vi "Correct Na-DAS_7609 sample interval error.vi"() -> ()   [LabVIEW 2022 SP3]
uses:
  Globals/Meas_global.vi
  Controls/Trigger_Mode.ctl
panel:
  out "Req Sample Rate Hz":dbl
  out "Delay Factor (s) per LDA sample":dbl
  in  "Apply time shift":bool=TRUE
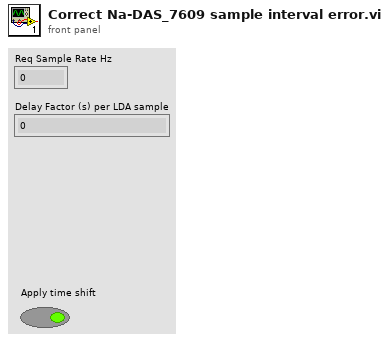
[diagram p1: front panel]
types:
  T1 = typedef "Time_Trace_Cluster.ctl" = cluster{"Weighting":dbl[], "Voltage":dbl[], "Eng Values":dbl[]}
  T2 = typedef "Trigger_Mode.ctl" = enum16{"Free Running", "Start on Trigger", "Trigger Every Block", "Trigger Every Sample"}
  T3 = typedef "Analysis_info_cluster.ctl" = cluster{"Colour":u32, "Inst type":T4, "Inst name":string, "Symbol":string, "Code name":string, "Extra Info":string, "Inst Array":T5, "Extra Titles":string[], "Extra Values":string[], "U":dbl, "u^2":dbl, "u^3":dbl, "u^4":dbl, "Skew_u":dbl, "Kurt_u":dbl, "Sd Error in Mean":dbl, "% u'/U":dbl, "X":dbl, "Y":dbl, "Z":dbl, "Timescale integral Estimate":dbl, "Sd Error in Variance":dbl, "Calib File":path, "Calib Constants":dbl[], "Output Position":bool, "Stats":enum16{"None", "Basic", "Full"}, "Av Sampling Rate":dbl, "Av No of Samples":dbl, "Total Meas Time (s)":dbl, "ADAM Ch Name":string, "Max value":dbl, "Min value":dbl, "Req Sample Rate Hz":dbl, "Sync Delay Time (s)":dbl, "Ch No":i16, "Device":string, "Use Latest Calib":bool, "Port":string, "Metadata Ch Names":string[], "Metadata Ch Values":string[], "Label":string}
  T4 = typedef "Inst_type.ctl" = enum16{"Raw voltage", "Raw with zero offsetting", "Propeller anemometer", "Pressure Transducer", "Pitot-static tube", "Hot wire", "Cross wire 1", "Cross wire 2", "Generic Linear", "Generic Polynomial", "Generic BackPoly", "Fast FID", "Thermocouple", "Cold wire", "Pulsed Wire", "LDA Vel", "LDA Tran time", "LDA Arr time", "Microphone"}
  T5 = typedef "Instrument_Array.ctl" = enum16{"PWA", "LDA", "Analogue"}
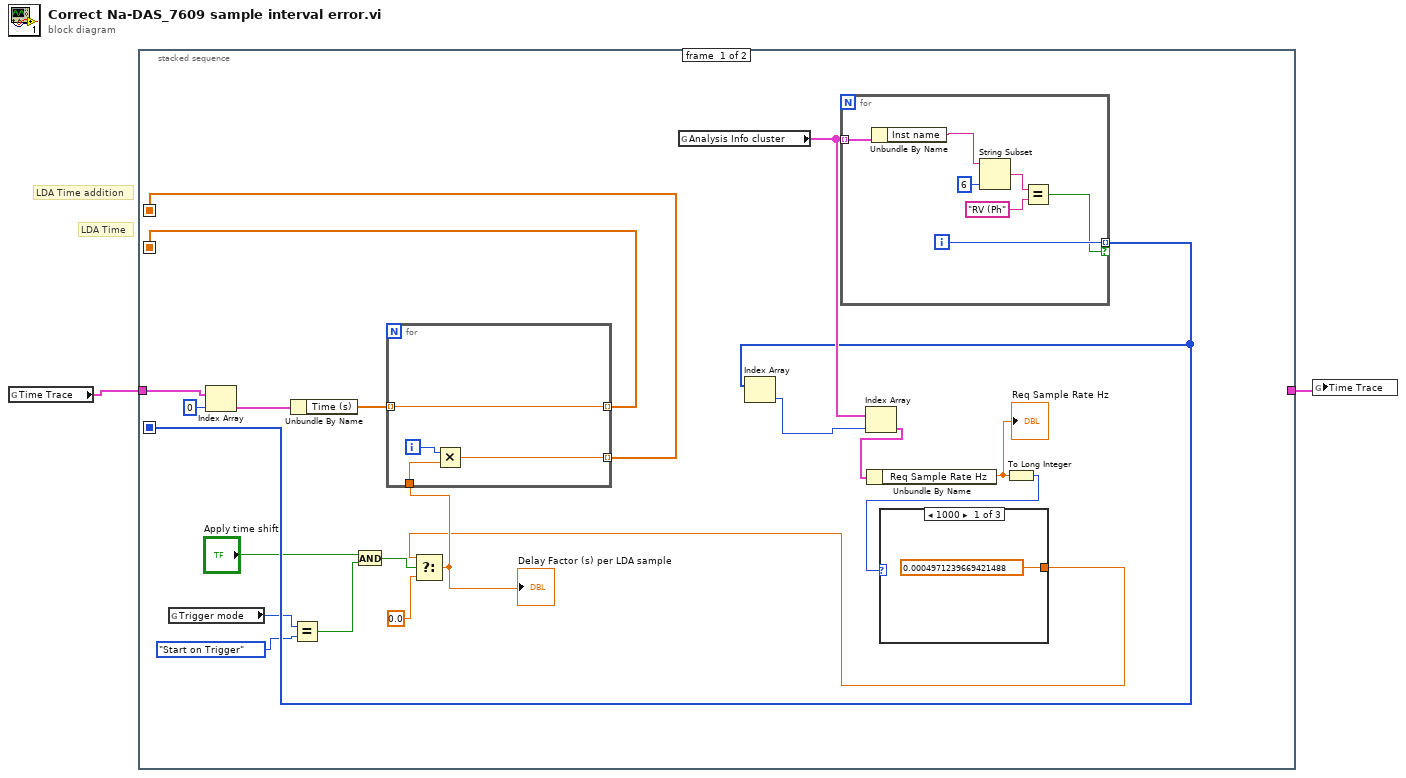
[diagram p0: block diagram]
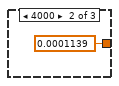
[diagram p2: hidden frame]
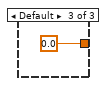
[diagram p3: hidden frame]
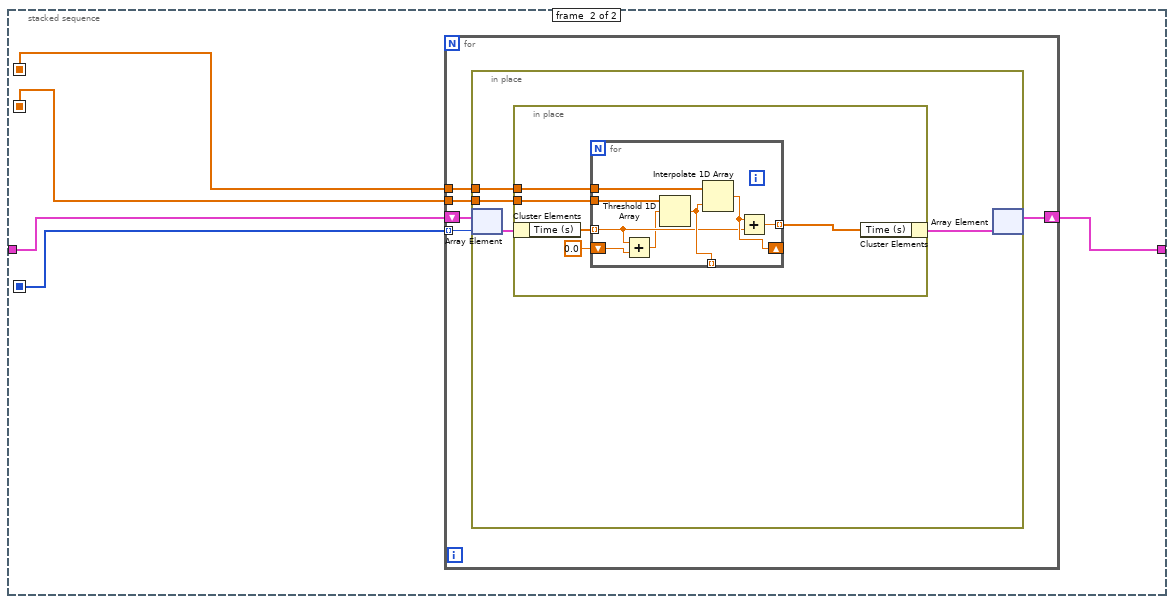
[diagram p4: hidden frame]
diagram:
  # "LDA Time addition"
  # "LDA Time"
  n1 = global read "Meas_global.vi" "Time Trace"() -> (w2:T1[])
  n2 = stacked-sequence {
    seq-local: [w18 _] -> [_ w38]
    seq-local: [w19 _] -> [_ w39]
    seq-local: [w9 _] -> [_ w37]
    tunnel: w2 -> [w22 w41]
    tunnel: [_ w40] -> w1
    frame #0 {
      n3 = global read "Meas_global.vi" "Trigger mode"() -> (w6:T2)
      n4 = Index Array(array=w22, index=0) -> (element=w20:T1)
      n5 = Unbundle By Name(w20) -> ("Time (s)"=w17:dbl[])
      n6 = Equal?(x=w6, y=Trigger_Mode."Start on Trigger" ("Trigger mode")) -> (x = y?=w4:bool)
      n7 = And(x="Apply time shift", y=w4) -> (x .and. y?=w5:bool)
      n8 = global read "Meas_global.vi" "Analysis Info cluster"() -> (w14:T3[])
      n9 = for {
        tunnel: w14 -> [w29] mode=indexing
        tunnel: [w27] -> w9 mode=indexing if=w26
        i -> [w27]
        n10 = Unbundle By Name(w29) -> ("Inst name"=w28:string)
        n11 = String Subset(string=w28, length (rest)=6 ("length (rest)")) -> (substring=w30:string)  [unwired: 1 out]
        n12 = Equal?(x=w30, y="RV (Ph") -> (x = y?=w26:bool)
      }
      n13 = Index Array(array=w9) -> (element=w8:i32)  [unwired: 1 in]
      n14 = Index Array(array=w14, index=w8) -> (element=w12:T3)
      n15 = Unbundle By Name(w12) -> ("Req Sample Rate Hz"=w11:dbl)
      "Req Sample Rate Hz" <- w11
      n16 = To Long Integer(number=w11) -> (32bit integer=w10:i32)
      n17 = case shown="1000" w10 {
        tunnel: [0.0004971239669421488 ("Factor 2") 0.0001139 ("Factor 2") 0.0 ("Factor 2")] -> w13
        frame 1000 {
        }
        frame 4000 {
        }
        frame Default {
        }
      }
      n18 = Select(t=w13, s=w5, f=0.0) -> (s? t:f=w15:dbl)
      "Delay Factor (s) per LDA sample" <- w15
      n19 = for {
        tunnel: w15 -> [w35]
        tunnel: [w34] -> w19 mode=indexing
        tunnel: [w33] -> w18 mode=indexing
        tunnel: w17 -> [w33] mode=indexing
        i -> [w36]
        n20 = Multiply(x=w36, y=w35) -> (x*y=w34:dbl)
      }
    }
    frame #1 {
      n21 = for {
        shift-right: [w44] -> w40
        shift-left: w41 -> [w46]
        tunnel: w37 -> [w45] mode=indexing
        tunnel: w38 -> [w43]
        tunnel: w39 -> [w42]
        n22 = in-place {
          in-place-border: w43 -> [w48]
          in-place-border: w42 -> [w47]
          n23 = in-place-array #1(w46, w45) -> (w50:T1)
          n24 = in-place {
            in-place-border: w48 -> [w55]
            in-place-border: w47 -> [w54]
            n25 = in-place-cluster #2(w50) -> ("Time (s)"=w53:dbl[])
            n26 = for {
              tunnel: w53 -> [w57] mode=indexing
              tunnel: w55 -> [w63]
              tunnel: w54 -> [w62]
              tunnel: [w61] -> w52 mode=indexing
              tunnel: [w60] -> _ mode=indexing
              shift-right: [w59] -> _
              shift-left: 0.0 -> [w58]
              n27 = Add(x=w57, y=w58) -> (x+y=w56:dbl)
              n28 = Threshold 1D Array(2:w56, 3:w63) -> (0:w60:dbl)  [unwired: 1 in]
              n29 = Interpolate 1D Array(1:w60, 2:w62) -> (0:w59:dbl)
              n30 = Add(x=w59, y=w57) -> (x+y=w61:dbl)
            }
            n31 = in-place-cluster #2("Time (s)"=w52) -> (w49:T1)
          }
          n32 = in-place-array #1(w49) -> (w44:T1[])  [unwired: 1 out]
        }
      }
    }
  }
  n33 = global write "Meas_global.vi" "Time Trace"(w1) -> ()
